vi "velocidade media.vi"(6 "Time Stamp 2":timestamp, 9 "x 2":dbl, 10 "Time Stamp 1":timestamp, 11 "x1":dbl) -> (3 "speed (cm/s)":dbl)   [LabVIEW 2016]
panel:
  # "CALCULA A VELOCIDADE EM cm/s\nAS ENTRADAS X DEVEM ESTAR EM mm"
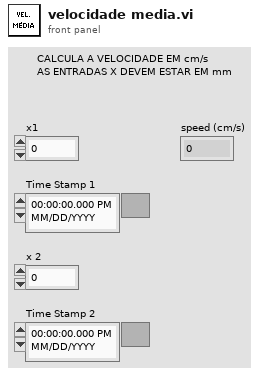
[diagram p1: front panel]
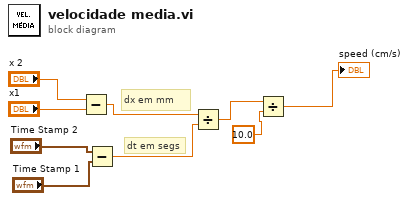
[diagram p0: block diagram]
diagram:
  # "dx em mm"
  # "dt em segs"
  n1 = Subtract(x="x 2", y="x1") -> (x-y=w5:dbl)
  n2 = Subtract(x="Time Stamp 2", y="Time Stamp 1") -> (x-y=w6:dbl)
  n3 = Divide(x=w5, y=w6) -> (x/y=w8:dbl)
  n4 = Divide(x=w8, y=10.0) -> (x/y=→"speed (cm/s)":dbl)
